vi "Simple TCP - Server.vi"() -> ()   [LabVIEW 2013]
doc: "演示设置基本TCP连接、建立连接后发送数据至指定端口并在完成发送后中止连接的方法。VI设计为TCP连接断开时停止。本范例中发送的数据为随机数数组。"
panel:
  in  "客户端关闭":string="客户端VI关闭了连接。"
  out "波形图":dbl[](graph)
  in  "停止":bool
  # "概述：演示使用TCP函数初始化可向客户端VI发送数据的TCP服务器。\n操作步骤：\n1. 运行VI。\n2. 打开Simple TCP - Client.vi并按前面板上的说明操作。注意，如运行本VI后执行该操作等待时间超过30秒，将发生超时。\n3. 单击停止可停止VI。注意，如停止客户端VI，该VI将自动停止。"
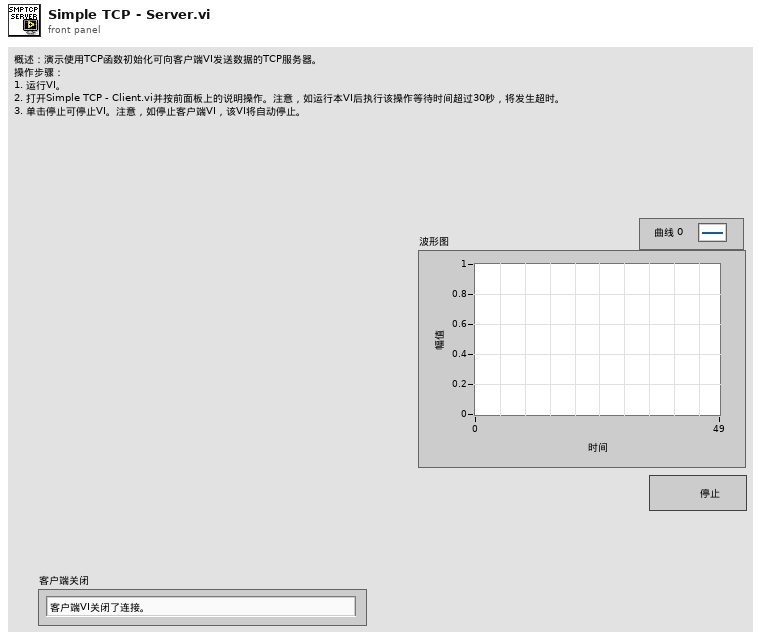
[diagram p1: front panel]
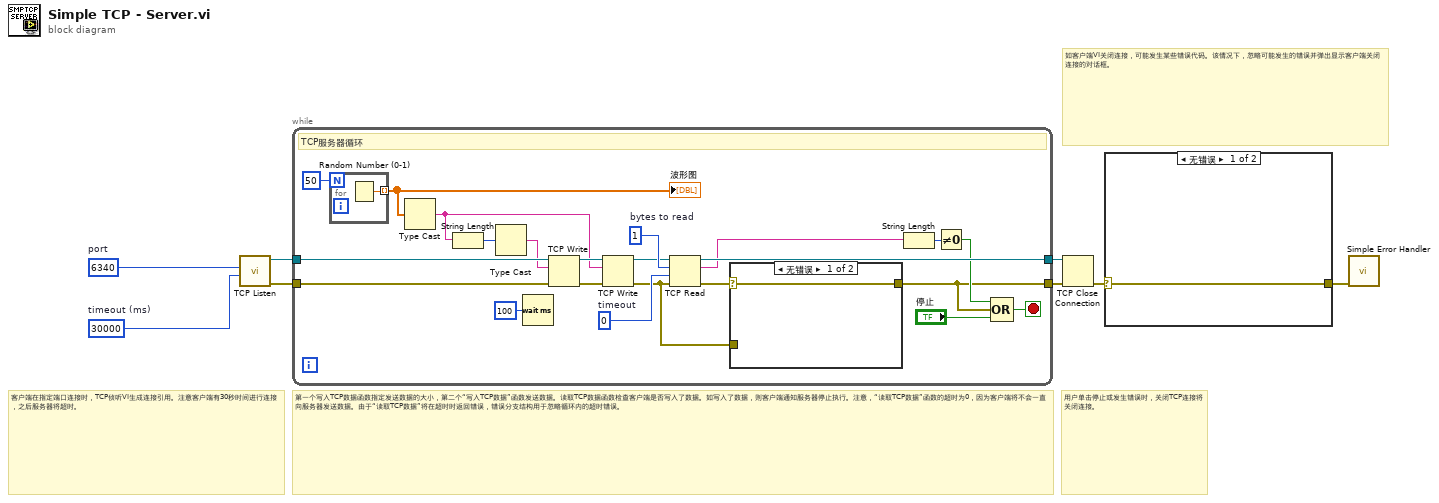
[diagram p0: block diagram]
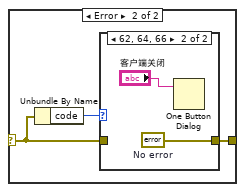
[diagram p2: hidden frame]
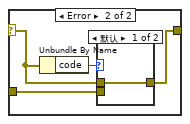
[diagram p4: hidden frame]
diagram:
  w1 = u16 6340  # port
  w2 = 30000  # timeout (ms)
  # "用户单击停止或发生错误时，关闭TCP连接将关闭连接。"
  # "客户端在指定端口连接时，TCP侦听VI生成连接引用。注意客户端有30秒时间进行连接，之后服务器将超时。"
  # "如客户端VI关闭连接，可能发生某些错误代码。该情况下，忽略可能发生的错误并弹出显示客户端关闭连接的对话框。"
  # "第一个写入TCP数据函数指定发送数据的大小，第二个“写入TCP数据”函数发送数据。读取TCP数据函数检查客户端是否写入了数据。如写入了数据，则客户端通知服务器停止执行。注意，“读取TCP数据”函数的超时为0，因为客户端将不会一直向服务器发送数据。由于“读取TCP数据”将在超时时返回错误，错误分支结构用于忽略循环内的超时错误。"
  n1 = call <vilib>:"TCP Listen.vi"("timeout ms (wait forever: -1)"=w2, "port"=w1) -> ("error out"=w3:errorcluster, "connection ID"=w4:refnum<k5>)  [unwired: 5 in, 3 out]
  n2 = while {
    tunnel: [w10] -> w7
    tunnel: [w16] -> w8
    tunnel: w4 -> [w30]
    tunnel: w3 -> [w21]
    stop <- w23 stop-if-true
    w15 = 0  # timeout
    w18 = 1  # bytes to read
    # "TCP服务器循环"
    n3 = for {
      N: 50 ("# of Points") -> [_]
      tunnel: [w38] -> w19 mode=indexing
      n4 = Random Number (0-1)() -> (number: 0 to 1=w38:dbl)
    }
    "波形图" <- w19
    n5 = Type Cast(x=w19) -> (*(type *) &x=w25:string)  [unwired: 1 out]
    n6 = String Length(string=w25) -> (length=w27:i32)
    n7 = Type Cast(x=w27) -> (*(type *) &x=w26:string)  [unwired: 1 out]
    n8 = Wait (ms)(milliseconds to wait=u32 100) -> ()  [unwired: 1 out]
    n9 = TCP Write(connection ID=w30, data in=w26, error in (no error)=w21) -> (connection ID out=w29:refnum<k5>, error out=w28:errorcluster)  [unwired: 2 out]
    n10 = TCP Write(connection ID=w29, data in=w25, error in (no error)=w28) -> (connection ID out=w17:refnum<k5>, error out=w9:errorcluster)  [unwired: 2 out]
    n11 = TCP Read(connection ID=w17, bytes to read=w18, error in (no error)=w9, 9:w15) -> (connection ID out=w16:refnum<k5>, data out=w13:string, error out=w11:errorcluster)  [unwired: 1 out]
    n12 = case shown="无错误" w11 {
      selector: w11 -> [w31 w34]
      tunnel: [w31 w32] -> w10
      tunnel: w9 -> [_ w33]
      frame No Error {
      }
      frame Error {
        n13 = Unbundle By Name(w34) -> ("code"=w35:i32)
        n14 = case shown="默认" w35 {
          tunnel: w34 -> [w36 _]
          tunnel: w33 -> [_ w37]
          tunnel: [w36 w37] -> w32
          frame Default {
          }
          frame 56 {
          }
        }
      }
    }
    n15 = String Length(string=w13) -> (length=w14:i32)
    n16 = Not Equal To 0?(x=w14) -> (x != 0?=w12:bool)
    n17 = Compound Arithmetic op=OR(w12, w10, "停止") -> (w23:bool)
  }
  n18 = TCP Close Connection(connection ID=w8, error in (no error)=w7) -> (error out=w6:errorcluster)  [unwired: 2 out]
  n19 = case shown="无错误" w6 {
    selector: w6 -> [w39 w41]
    tunnel: [w39 w40] -> w5
    frame No Error {
    }
    frame Error {
      n20 = Unbundle By Name(w41) -> ("code"=w42:i32)
      n21 = case shown="62, 64, 66" w42 {
        tunnel: w41 -> [w43 _]
        tunnel: [w43 w45] -> w40
        frame Default {
        }
        frame 62, 64, 66 {
          w45 = errorcluster {"status"=FALSE, "code"=0, "source"=""}  # No error
          n22 = One Button Dialog(message="客户端关闭") -> ()  [unwired: 1 in, 1 out]
        }
      }
    }
  }
  n23 = call <vilib>:"Simple Error Handler.vi"("error in (no error)"=w5) -> ()  [unwired: 1 in, 8 out]
